vi "Sensor_limit_Ld.vi"(9 "d":dbl, 10 "PV":dbl, 11 "Limit L":dbl) -> (1 "Off":bool, 2 "On":bool, 3 "NaN":bool)   [LabVIEW 2019, in "Inputs.lvlib"]
uses:
  Inputs.lvlib
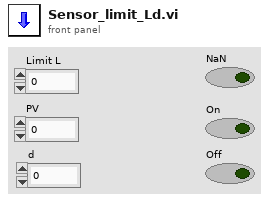
[diagram p1: front panel]
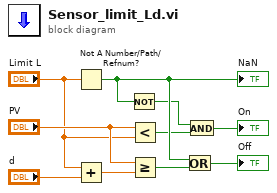
[diagram p0: block diagram]
diagram:
  n1 = Not A Number/Path/Refnum?(number/path/refnum="Limit L") -> (NaN/Path/Refnum?=w8:bool)
  "NaN" <- w8
  n2 = Add(x="Limit L", y="d") -> (x+y=w1:dbl)
  n3 = Not(x=w8) -> (.not. x?=w6:bool)
  n4 = Less?(x="PV", y="Limit L") -> (x < y?=w2:bool)
  n5 = Greater Or Equal?(x="PV", y=w1) -> (x >= y?=w3:bool)
  n6 = Or(x=w8, y=w3) -> (x .or. y?=→"Off":bool)
  n7 = And(x=w6, y=w2) -> (x .and. y?=→"On":bool)
